vi "Cube Drop.vi"   [LabVIEW 2020, in "VolatusDAQ.lvlib"]
uses:
  VolatusDAQ.lvlib
  DAQmxAI/DAQmxAI.lvclass
  DAQmxAO/DAQmxAO.lvclass
  DAQmxDI/DAQmxDI.lvclass
  DAQmxDO/DAQmxDO.lvclass
  VolatusData/VolatusData.lvlib
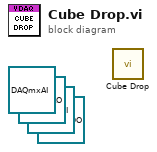
[diagram p0: block diagram]
diagram:
  (unwired) refnum<class "DAQmxDO.lvclass"> refnum ("VolatusDAQ.lvlib:DAQmxDO.lvclass")
  (unwired) refnum<class "DAQmxDI.lvclass"> refnum ("VolatusDAQ.lvlib:DAQmxDI.lvclass")
  (unwired) refnum<class "DAQmxAO.lvclass"> refnum ("VolatusDAQ.lvlib:DAQmxAO.lvclass")
  (unwired) refnum<class "DAQmxAI.lvclass"> refnum ("VolatusDAQ.lvlib:DAQmxAI.lvclass")
  n1 = call "Cube Drop.vi"() -> ()  [unwired: 12 in]
